vi "Integration Query.vi"(8 "error in (no error)":errorcluster, 10 "Element":u8=1 min=1 max=6 step=1, 11 "Yokogawa WT500 in":refnum<class "Yokogawa WT500.lvclass">) -> (0 "error out":errorcluster, 1 "Integration State":T1, 3 "Yokogawa WT500 out":refnum<class "Yokogawa WT500.lvclass">)   [LabVIEW 2013, in "Universal Power Meter.lvlib" / "Yokogawa WT500.lvlib" / "Yokogawa WT500.lvclass"]
uses:
  Yokogawa WT500.lvclass
  Universal Power Meter class/Integration State.ctl
  Universal Power Meter class/Universal Power Meter.lvclass
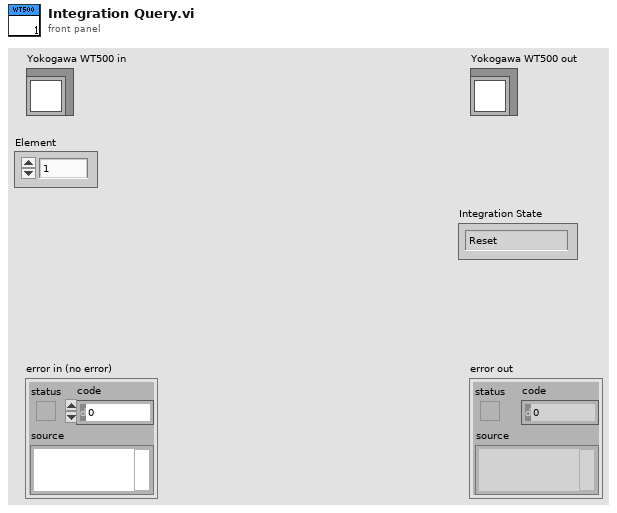
[diagram p1: front panel]
types:
  T1 = typedef "Universal Power Meter.lvlib/Universal Power Meter.lvclass/Integration State.ctl" = enum16{"Reset", "Stop", "Start"}
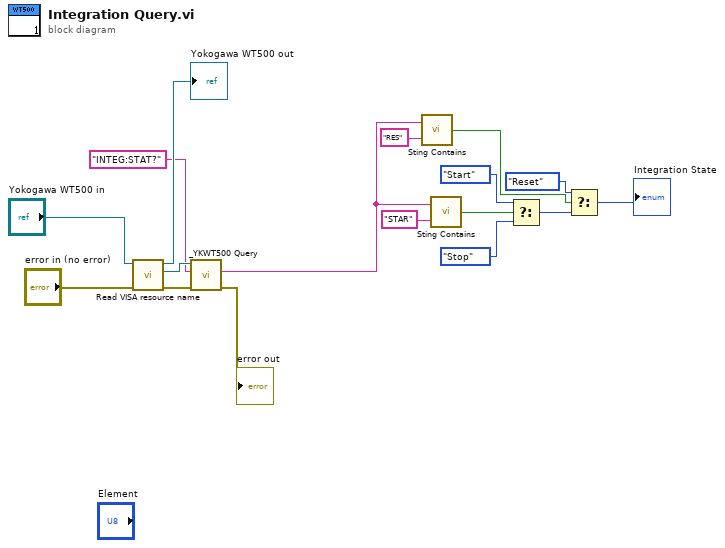
[diagram p0: block diagram]
diagram:
  n1 = call-dynamic "Read VISA resource name.vi"("error in (no error)"="error in (no error)", "Generic Instrument in"="Yokogawa WT500 in") -> ("error out"=w3:errorcluster, "VISA resource name"=w5:refnum<visa-resource-name>, "Generic Instrument out"=→"Yokogawa WT500 out":refnum<class "Yokogawa WT500.lvclass">)  [unwired: 7 in]
  n2 = call <instrlib>:"_YKWT500 Query.vi"("error in (no error)"=w3, "Write Data"="INTEG:STAT?", "VISA resource name"=w5) -> ("error out"=→"error out":errorcluster, "Read Data"=w1:string)  [unwired: 5 in, 2 out]
  n3 = call "Sting Contains.vi"("Expression to evaluate"="RES", "Input String"=w1) -> ("Boolean"=w13:bool)
  n4 = call "Sting Contains.vi"("Expression to evaluate"="STAR", "Input String"=w1) -> ("Boolean"=w11:bool)
  n5 = Select(t=Integration_State."Start" ("Integration State"), s=w11, f=Integration_State."Stop" ("Integration State")) -> (s? t:f=w10:T1)
  n6 = Select(t=Integration_State."Reset" ("Integration State"), s=w13, f=w10) -> (s? t:f=→"Integration State":T1)
